vi "main.vi"() -> (0 "Cancel":bool)   [LabVIEW 2014]
uses:
  <vilib>/Utility/file.llb/Read From Spreadsheet File (string).vi
  <vilib>/Utility/file.llb/Write To Spreadsheet File (string).vi
panel:
  out "Write file path":path=path "C:/Users/asus/Desktop/labview_final_project/program file/text data/member_list.txt"
  out "Read file path":path=path "C:/Users/asus/Desktop/labview_final_project/program file/text data/member_list.txt"
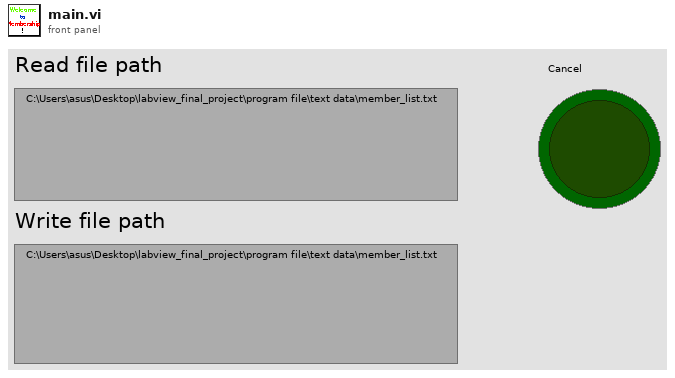
[diagram p1: front panel]
types:
  T1 = enum16{"User_data_input", "Is username empty?", "Is username used?", "Is password empty?", "Is password check pass?", "Input data"}
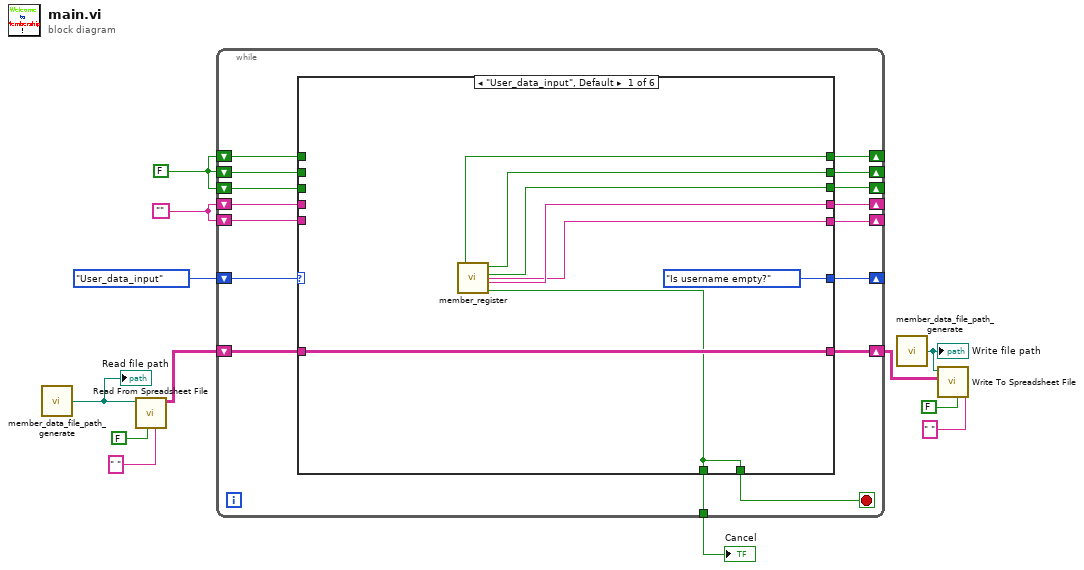
[diagram p0: block diagram]
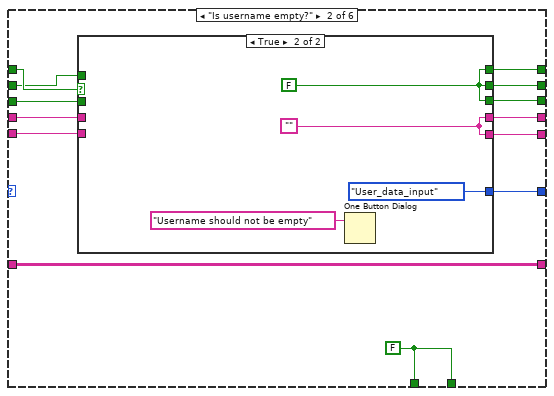
[diagram p2: hidden frame]
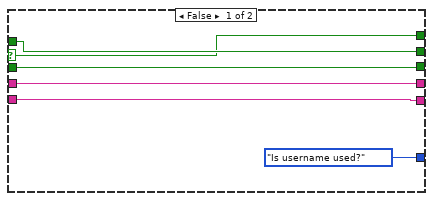
[diagram p3: hidden frame]
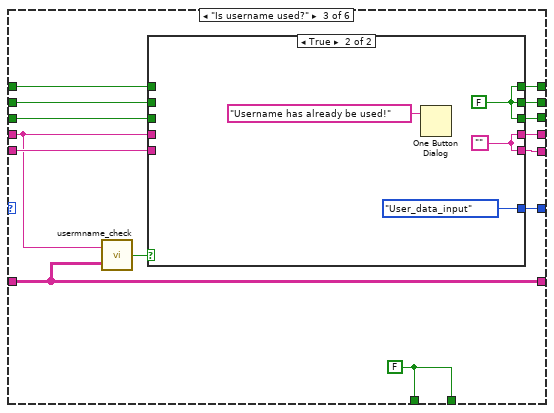
[diagram p4: hidden frame]
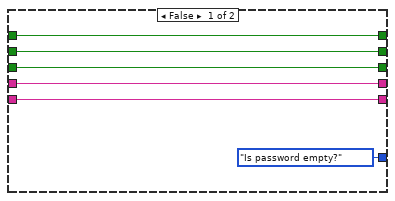
[diagram p5: hidden frame]
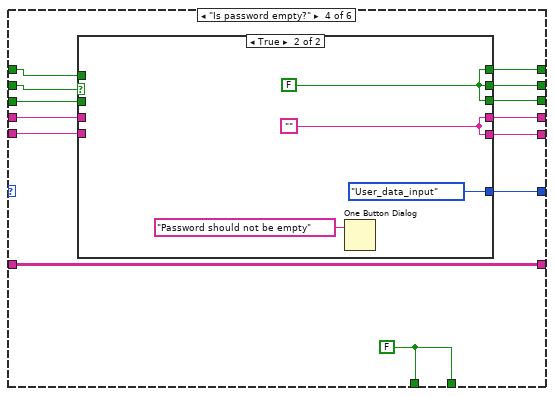
[diagram p6: hidden frame]
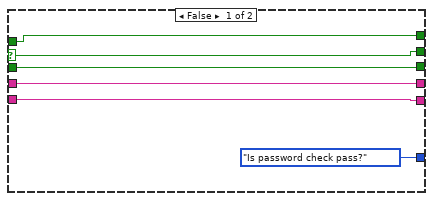
[diagram p7: hidden frame]
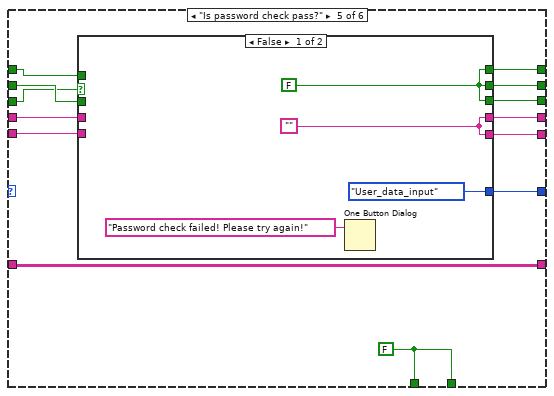
[diagram p8: hidden frame]
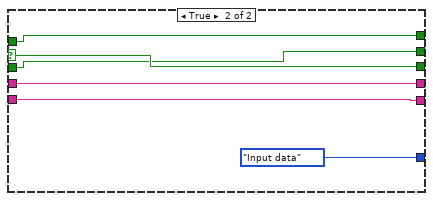
[diagram p9: hidden frame]
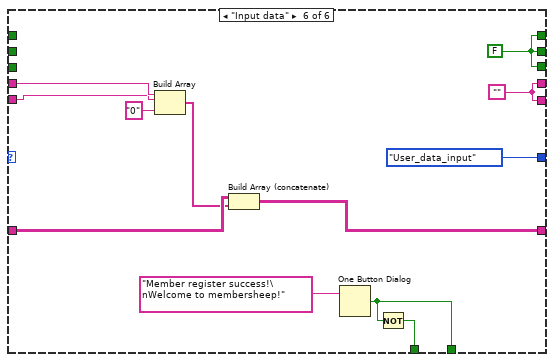
[diagram p10: hidden frame]
diagram:
  w10 = ""
  w11 = FALSE
  n1 = call "member_data_file_path_generate.vi"() -> ("appended path"=w2:path)
  "Read file path" <- w2
  n2 = call-poly <vilib>:"Read From Spreadsheet File.vi"("delimiter (\\t)"=" ", "transpose (no:F)"=FALSE, "file path (dialog if empty)"=w2) -> ("all rows"=w8:string[][])  [unwired: 4 in, 4 out]
  n3 = while {
    shift-right: [w27] -> _
    shift-left: T1."User_data_input" -> [w28]
    shift-right: [w26] -> _
    shift-left: w11 -> [w21]
    shift-right: [w25] -> _
    shift-left: w11 -> [w20]
    shift-right: [w24] -> _
    shift-left: w11 -> [w19]
    shift-right: [w23] -> _
    shift-left: w10 -> [w18]
    shift-right: [w22] -> _
    shift-left: w10 -> [w17]
    shift-right: [w15] -> w7
    shift-left: w8 -> [w16]
    tunnel: [w13] -> w3
    stop <- w14 stop-if-true
    n4 = case shown="\"User_data_input\", Default" w28 {
      tunnel: [T1."Is username empty?" w44 w62 w93 w117 T1."User_data_input"] -> w27
      tunnel: [w35 w43 w68 w92 w116 w134] -> w26
      tunnel: [w34 w42 w67 w91 w115 w134] -> w25
      tunnel: [w33 w41 w66 w90 w114 w134] -> w24
      tunnel: [w32 w40 w64 w89 w113 w133] -> w23
      tunnel: [w31 w39 w65 w88 w112 w133] -> w22
      tunnel: w21 -> [_ w49 w69 w86 w111 _]
      tunnel: w20 -> [_ w48 w70 w87 w110 _]
      tunnel: w19 -> [_ w47 w71 w96 w109 _]
      tunnel: w18 -> [_ w46 w63 w95 w119 w140]
      tunnel: w17 -> [_ w45 w72 w94 w118 w139]
      tunnel: [w29 w37 w60 w84 w107 w131] -> w14
      tunnel: w16 -> [w30 w38 w61 w85 w108 w137]
      tunnel: [w30 w38 w61 w85 w108 w135] -> w15
      tunnel: [w29 w37 w60 w84 w107 w130] -> w13
      frame "User_data_input", Default {
        n5 = call "member_register.vi"() -> ("Cancel"=w29:bool, "Username out"=w32:string, "Password check pass"=w33:bool, "Password empty"=w34:bool, "Password out"=w31:string, "Username empty"=w35:bool)
      }
      frame "Is username empty?" {
        w37 = FALSE
        n6 = case shown="True" w49 {
          selector: w49 -> [w51 _]
          tunnel: w48 -> [w55 _]
          tunnel: w47 -> [w54 _]
          tunnel: w46 -> [w53 _]
          tunnel: w45 -> [w52 _]
          tunnel: [T1."Is username used?" T1."User_data_input"] -> w44
          tunnel: [w51 w57] -> w43
          tunnel: [w55 w57] -> w42
          tunnel: [w54 w57] -> w41
          tunnel: [w53 w56] -> w40
          tunnel: [w52 w56] -> w39
          frame False {
          }
          frame True {
            w56 = ""
            w57 = FALSE
            n7 = One Button Dialog(message="Username should not be empty") -> ()  [unwired: 1 in, 1 out]
          }
        }
      }
      frame "Is username used?" {
        w60 = FALSE
        n8 = call "usermname_check.vi"("first row"=w61, "String"=w63) -> ("Boolean"=w73:bool)
        n9 = case shown="True" w73 {
          tunnel: w72 -> [w76 _]
          tunnel: w71 -> [w77 _]
          tunnel: w70 -> [w78 _]
          tunnel: w69 -> [w79 _]
          tunnel: [w79 w83] -> w68
          tunnel: [w78 w83] -> w67
          tunnel: [w77 w83] -> w66
          tunnel: [w76 w82] -> w65
          tunnel: [w75 w82] -> w64
          tunnel: w63 -> [w75 _]
          tunnel: [T1."Is password empty?" T1."User_data_input"] -> w62
          frame False {
          }
          frame True {
            w82 = ""
            w83 = FALSE
            n10 = One Button Dialog(message="Username has already be used!") -> ()  [unwired: 1 in, 1 out]
          }
        }
      }
      frame "Is password empty?" {
        w84 = FALSE
        n11 = case shown="True" w87 {
          selector: w87 -> [w98 _]
          tunnel: w86 -> [w97 _]
          tunnel: w96 -> [w102 _]
          tunnel: w95 -> [w101 _]
          tunnel: w94 -> [w100 _]
          tunnel: [T1."Is password check pass?" T1."User_data_input"] -> w93
          tunnel: [w97 w104] -> w92
          tunnel: [w98 w104] -> w91
          tunnel: [w102 w104] -> w90
          tunnel: [w101 w103] -> w89
          tunnel: [w100 w103] -> w88
          frame False {
          }
          frame True {
            w103 = ""
            w104 = FALSE
            n12 = One Button Dialog(message="Password should not be empty") -> ()  [unwired: 1 in, 1 out]
          }
        }
      }
      frame "Is password check pass?" {
        w107 = FALSE
        n13 = case shown="False" w109 {
          selector: w109 -> [_ w125]
          tunnel: w111 -> [_ w126]
          tunnel: w110 -> [_ w124]
          tunnel: w119 -> [_ w129]
          tunnel: w118 -> [_ w128]
          tunnel: [T1."User_data_input" T1."Input data"] -> w117
          tunnel: [w121 w126] -> w116
          tunnel: [w121 w124] -> w115
          tunnel: [w121 w125] -> w114
          tunnel: [w120 w129] -> w113
          tunnel: [w120 w128] -> w112
          frame False {
            w120 = ""
            w121 = FALSE
            n14 = One Button Dialog(message="Password check failed! Please try again!") -> ()  [unwired: 1 in, 1 out]
          }
          frame True {
          }
        }
      }
      frame "Input data" {
        w133 = ""
        w134 = FALSE
        n15 = Build Array(w140, w139, "0") -> (w136:string[])
        n16 = Build Array (concatenate)(w137, w136) -> (w135:string[][])
        n17 = One Button Dialog(message="Member register success!\nWelcome to membersheep!") -> (true=w131:bool)  [unwired: 1 in]
        n18 = Not(x=w131) -> (.not. x?=w130:bool)
      }
    }
  }
  "Cancel" <- w3
  n19 = call "member_data_file_path_generate.vi"() -> ("appended path"=w1:path)
  "Write file path" <- w1
  n20 = call-poly <vilib>:"Write To Spreadsheet File.vi"("delimiter (\\t)"=" ", "transpose? (no:F)"=FALSE, "2D data"=w7, "file path (dialog if empty)"=w1) -> ()  [unwired: 4 in, 1 out]
